vi "HS256.vi"   [LabVIEW 2020]
uses:
  Crypto/Signatures/HMAC/HMAC.lvclass
  Crypto/Hashes/SHA-256/SHA-256.lvclass
  C:/dev/LabVIEW/IlluminatedG/lv-web-crypto/lv-crypto/Crypto/Hash/Hash.lvclass
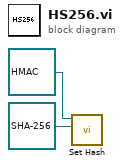
[diagram p0: block diagram]
diagram:
  n1 = call "Set Hash.vi"("Hash"=refnum<class "SHA-256.lvclass"> refnum ("Crypto.lvlib:SHA-256.lvclass"), "HMAC in"=refnum<class "HMAC.lvclass"> refnum ("Crypto.lvlib:HMAC.lvclass")) -> ()  [unwired: 8 in, 2 out]
